vi "_Add Device.vi"(8 "error in (no error)":errorcluster, 10 "Device":refnum<class "Device.lvclass">, 11 "DeviceListPanel in":refnum<class "DeviceListPanel.lvclass">) -> (0 "error out":errorcluster, 3 "DeviceListPanel out":refnum<class "DeviceListPanel.lvclass">)   [LabVIEW 2020, in "PicoG-App.lvlib" / "DeviceListPanel.lvclass"]
uses:
  DeviceListPanel.lvclass
  Device/Device.lvclass
  DeviceListPanel.lvclass/DeviceListPanel.ctl
  DeviceArrayPanel/DeviceArrayPanel.lvclass
  C:/Program Files (x86)/National Instruments/LabVIEW 2020/vi.lib/IlluminatedG/IG OOPanel/OOPanel/ArrayPanel/ArrayPanel.lvclass
  Device and Panel.ctl
  <vilib>/IlluminatedG/IG OOPanel/OOPanel/ArrayManager/ArrayManager.lvclass
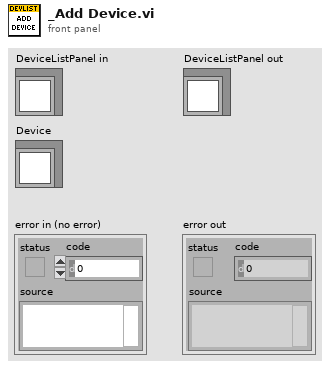
[diagram p1: front panel]
types:
  T1 = typedef "PicoG-App.lvlib/Device.lvclass/Device Key.ctl" = cluster{"Platform":string, "Board":string, "ID":string}
  T2 = typedef "PicoG-App.lvlib/DeviceListPanel.lvclass/Device and Panel.ctl" = cluster{"Device":refnum<class "Device.lvclass">, "Panel":refnum<class "DeviceArrayPanel.lvclass">}
  T3 = typedef "PicoG-App.lvlib/DeviceListPanel.lvclass/Ref Data.ctl" = cluster{"Map":map{T1, T2}}
  T4 = typedef "PicoG-App.lvlib/DeviceListPanel.lvclass/Device Update Action.ctl" = enum16{"Ignore", "Update", "Show Existing"}
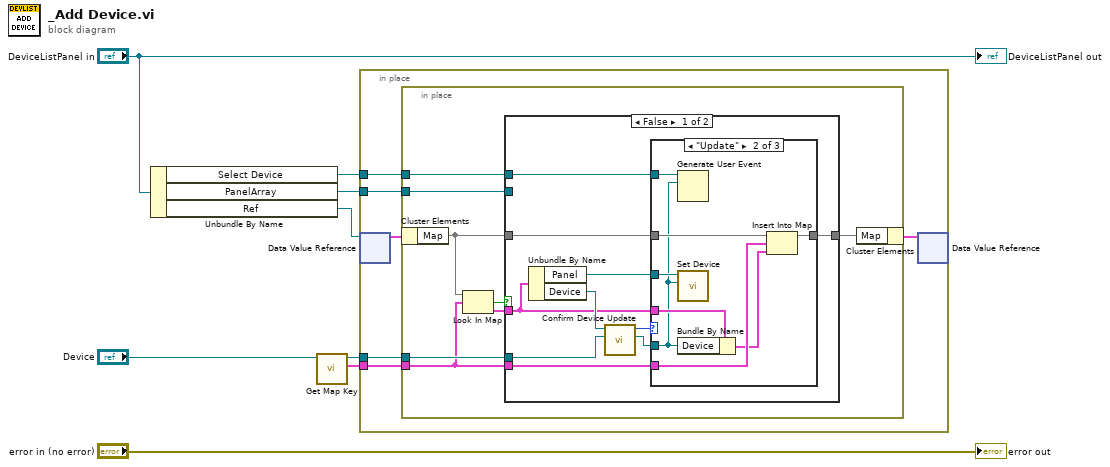
[diagram p0: block diagram]
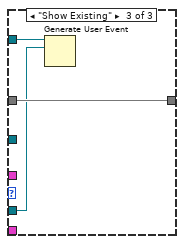
[diagram p3: hidden frame]
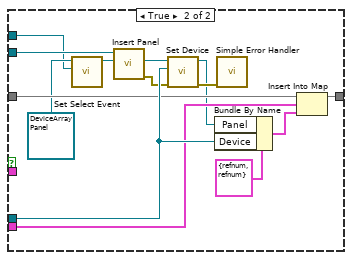
[diagram p4: hidden frame]
diagram:
  n1 = Unbundle By Name("DeviceListPanel in") -> ("Select Device"=w1:refnum<user-event>, "PanelArray"=w2:refnum<class "ArrayManager.lvclass">, "Ref"=w7:refnum<data-value>)
  n2 = call "Get Map Key.vi"("Device in"="Device") -> ("Key"=w3:T1, "Device out"=w4:refnum<class "Device.lvclass">)  [unwired: 8 in, 1 out]
  n3 = in-place {
    in-place-border: w4 -> [w12]
    in-place-border: w3 -> [w11]
    in-place-border: w2 -> [w10]
    in-place-border: w1 -> [w9]
    n4 = in-place-dvr #1(w7) -> (w14:T3)  [unwired: 1 out]
    n5 = in-place {
      in-place-border: w12 -> [w20]
      in-place-border: w11 -> [w17]
      in-place-border: w10 -> [w19]
      in-place-border: w9 -> [w15]
      n6 = in-place-cluster #2(w14) -> ("Map"=w21:map{T1, T2})
      n7 = Look In Map(map=w21, key=w17) -> (key not found?=w22:bool, value=w16:T2)  [unwired: 1 in]
      n8 = case shown="False" w22 {
        tunnel: w21 -> [w29 w54]
        tunnel: w20 -> [w31 w55]
        tunnel: w19 -> [_ w57]
        tunnel: [w28 w53] -> w18
        tunnel: w17 -> [w26 w51]
        tunnel: w16 -> [w27 _]
        tunnel: w15 -> [w23 w45]
        frame False {
          n9 = Unbundle By Name(w27) -> ("Panel"=w24:refnum<class "DeviceArrayPanel.lvclass">, "Device"=w32:refnum<class "Device.lvclass">)
          n10 = call "Confirm Device Update.vi"("Updated Device"=w31, "Existing Device"=w32) -> ("Device"=w25:refnum<class "Device.lvclass">, "Result"=w30:T4)  [unwired: 8 in]
          n11 = case shown="\"Update\"" w30 {
            tunnel: w29 -> [w33 w39 w44]
            tunnel: [w33 w38 w44] -> w28
            tunnel: w27 -> [_ w41 _]
            tunnel: w26 -> [_ w37 _]
            tunnel: w25 -> [_ w34 w42]
            tunnel: w24 -> [_ w40 _]
            tunnel: w23 -> [_ w35 w43]
            frame "Ignore" {
            }
            frame "Update" {
              n12 = Generate User Event(user event=w35, event data cluster=w34) -> ()  [unwired: 2 in, 2 out]
              n13 = call "Set Device.vi"("Device"=w34, "DeviceArrayPanel in"=w40) -> ()  [unwired: 8 in, 2 out]
              n14 = Bundle By Name(cluster=w41, "Device"=w34) -> (w36:T2)
              n15 = Insert Into Map(map in=w39, key=w37, value=w36) -> (map out=w38:map{T1, T2})  [unwired: 2 out]
            }
            frame "Show Existing" {
              n16 = Generate User Event(user event=w43, event data cluster=w42) -> ()  [unwired: 2 in, 2 out]
            }
          }
        }
        frame True {
          n17 = call "Set Select Event.vi"("Select Event"=w45, "DeviceArrayPanel in"=refnum<class "DeviceArrayPanel.lvclass"> refnum ("PicoG-App.lvlib:DeviceArrayPanel.lvclass")) -> ("DeviceArrayPanel out"=w46:refnum<class "DeviceArrayPanel.lvclass">)  [unwired: 8 in, 1 out]
          n18 = call <vilib>:"Insert Panel.vi"("Panel/Type"=w46, "PanelArray in"=w57) -> ("error out"=w48:errorcluster, "Panel"=w49:refnum<class "DeviceArrayPanel.lvclass">)  [unwired: 7 in, 1 out]
          n19 = call "Set Device.vi"("error in (no error)"=w48, "Device"=w55, "DeviceArrayPanel in"=w49) -> ("error out"=w58:errorcluster, "DeviceArrayPanel out"=w50:refnum<class "DeviceArrayPanel.lvclass">)  [unwired: 7 in]
          n20 = Bundle By Name(cluster=T2 {"Device"=refnum, "Panel"=refnum} ("Device and Panel"), "Panel"=w50, "Device"=w55) -> (w52:T2)
          n21 = call <vilib>:"Simple Error Handler.vi"("error in (no error)"=w58) -> ()  [unwired: 4 in, 5 out]
          n22 = Insert Into Map(map in=w54, key=w51, value=w52) -> (map out=w53:map{T1, T2})  [unwired: 2 out]
        }
      }
      n23 = in-place-cluster #2("Map"=w18) -> (w13:T3)
    }
    n24 = in-place-dvr #1(w13) -> ()  [unwired: 2 out]
  }
  "error out" <- "error in (no error)"
  "DeviceListPanel out" <- "DeviceListPanel in"
